vi "Open and Configure Scope Session.vi"(7 "Channels":string="0" caption="channels", 8 "error in":errorcluster, 9 "Vertical range":dbl=10.0 caption="vertical range" format="%.2f", 10 "Sample rate":dbl=20000000.0 caption="min sample rate" format="%^.2e", 11 "Scope resource":refnum<k15>="6571" caption="resource name") -> (0 "error out":errorcluster, 3 "Scope seesion out":refnum<k15>)   [LabVIEW 2021]
uses:
  <instrlib>/niScope/Controls/niScope trigger source digital.ctl
  <instrlib>/niScope/Configure/Trigger/niScope Configure Trigger Digital.vi
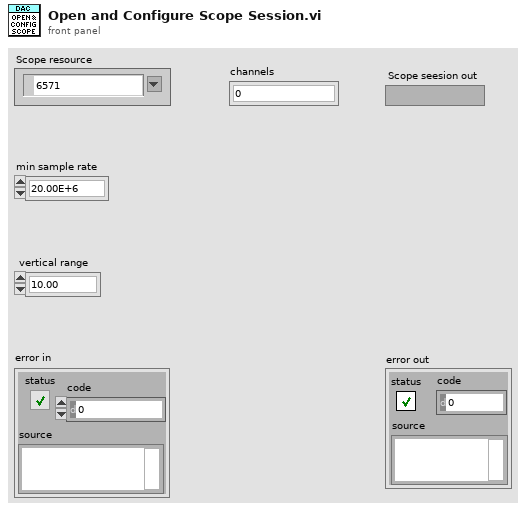
[diagram p1: front panel]
types:
  T1 = typedef "niScope trigger source digital.ctl" = string
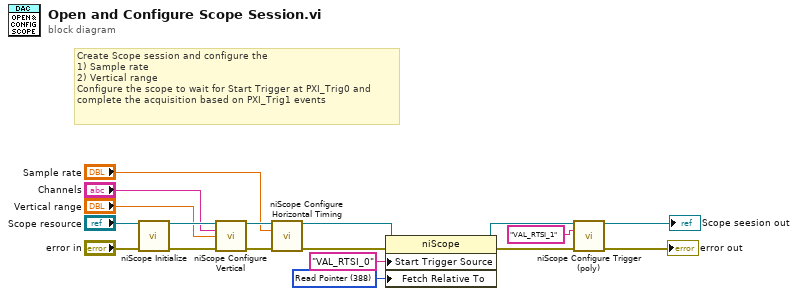
[diagram p0: block diagram]
diagram:
  w3 = 388 items=["Start"=482, "Trigger"=483, "Pretrigger"=477, "Now"=481, "Read Pointer"=388] ("Fetch:Fetch Relative To")
  # "Create Scope session and configure the \n1) Sample rate\n2) Vertical range\nConfigure the scope to wait for Start Trigger at PXI_Trig0 and \ncomplete the acquisition based on PXI_Trig1 events"
  n1 = call <instrlib>:"niScope Initialize.vi"("resource name"="Scope resource", "error in"="error in") -> ("instrument handle"=w16:refnum<k15>, "error out"=w15:errorcluster)  [unwired: 12 in]
  n2 = call <instrlib>:"niScope Configure Vertical.vi"("instrument handle"=w16, "channels"="Channels", "vertical range"="Vertical range", "error in"=w15) -> ("instrument handle out"=w12:refnum<k15>, "error out"=w11:errorcluster)  [unwired: 10 in]
  n3 = call <instrlib>:"niScope Configure Horizontal Timing.vi"("instrument handle"=w12, "min sample rate"="Sample rate", "error in"=w11) -> ("instrument handle out"=w8:refnum<k15>, "error out"=w9:errorcluster)  [unwired: 11 in]
  n4 = property class="niScope"(reference=w8, error in=w9, "Start Trigger Source"="VAL_RTSI_0" ("Synchronization:Start Trigger (Acq. Arm): Source"), "Fetch Relative To"=w3) -> (reference out=w5:refnum<k15>, error out=w6:errorcluster)
  n5 = call-poly <instrlib>:"niScope Configure Trigger (poly).vi"("instrument handle"=w5, "trigger source"=T1 "VAL_RTSI_1", "error in"=w6) -> ("instrument handle out"=→"Scope seesion out":refnum<k15>, "error out"=→"error out":errorcluster)  [unwired: 11 in]
